vi "cliente_planta.vi"() -> ()   [LabVIEW 2023]
panel:
  in  "porta":dbl
  in  "agua cm3/s":dbl(slide) scale=0.0..500.0
  in  "barita g/s":dbl(slide) scale=0.0..1000.0
  out "DENSIDADE E SET POINT":cluster{dbl, "Setpoint":dbl}(graph)
  out "Numeric":dbl
  in  "ON/ OFF":bool
  out "DOSAGEM mA":string
  out "bytes escritos":i32
  out "corrente mA":string
  out "tipo de dosagem":string
  in  "Setpoint":dbl(slide) scale=0.8..1.4
  out "dado enviado para o servidor":string
  out "indicador de set point":string
  out "indicador de densidade":string
  in  "parametro a":dbl format="%#_13g"
  in  "parametro b":dbl format="%#_13g"
  in  "parametro c":dbl format="%#_13g"
  out "densidadeA":dbl
  out "SINAL DE CONTROLE AGUA":dbl(graph)
  out "Q1":dbl
  out "densidadeB":dbl
  out "SINAL DE CONTROLE BARITA":dbl(graph)
  in  "A":dbl=0.1 format="%#_13g"
  in  "B":dbl=0.2 format="%#_13g"
  in  "C":dbl format="%#_13g"
  out "W2":dbl
  # "MODELO/BARITA"
  # "MODELO/ÁGUA"
  # "SAÍDA DO CLIENTE/ENTRADA DO CONTROLADOR"
  # "SAÍDA DO SERVIDOR/AÇÃO DE CONTROLE"
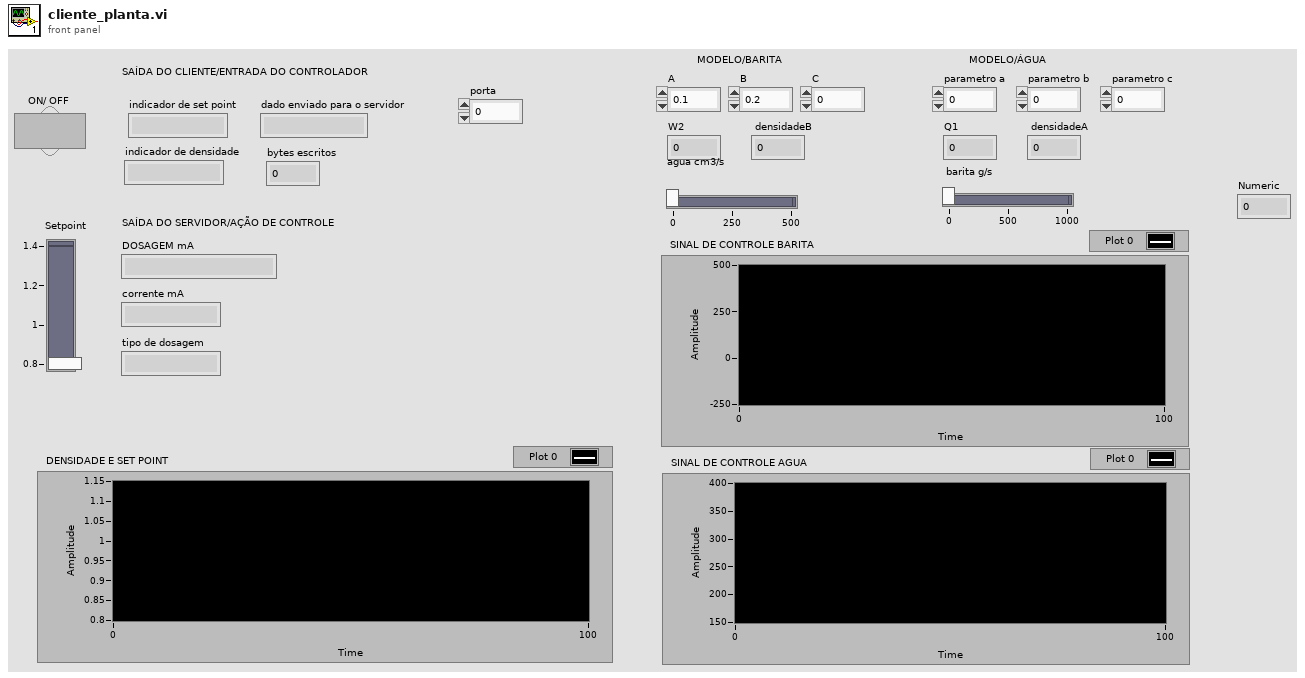
[diagram p1: front panel]
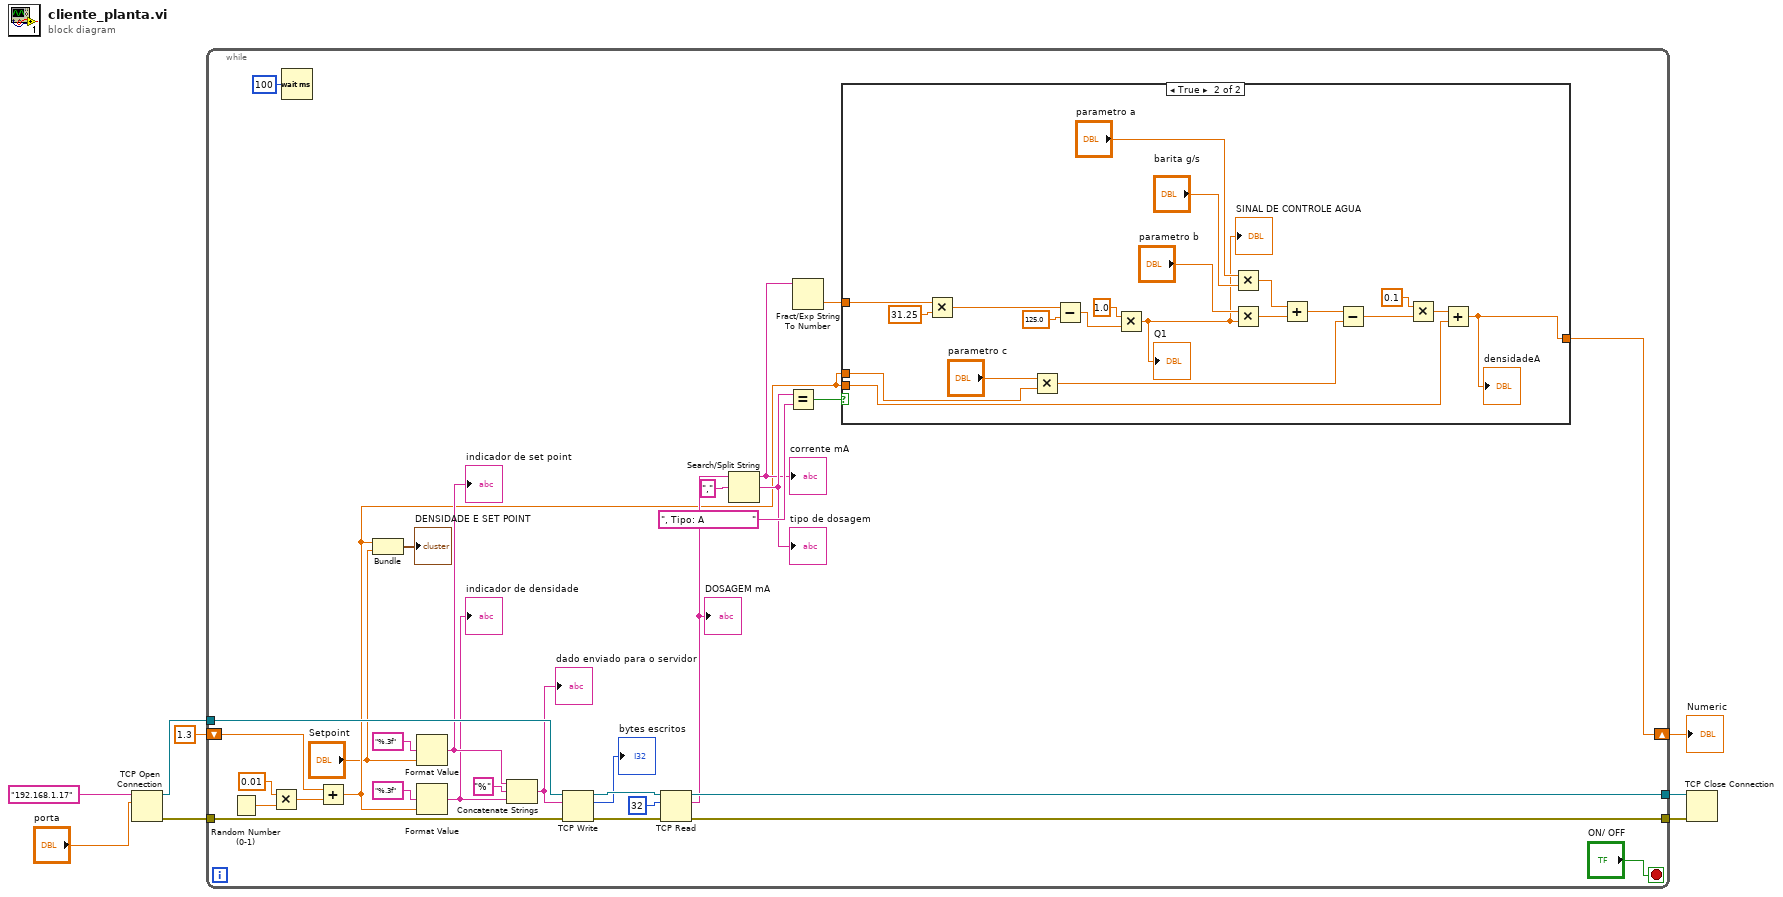
[diagram p0: block diagram]
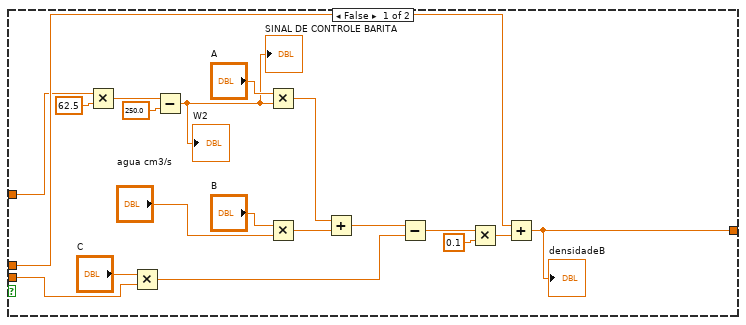
[diagram p2: hidden frame]
diagram:
  n1 = TCP Open Connection(address="192.168.1.17", remote port or service name="porta") -> (connection ID=w7:refnum<k5>, error out=w6:errorcluster)  [unwired: 3 in]
  n2 = while {
    tunnel: w7 -> [w37]
    tunnel: w6 -> [w36]
    tunnel: [w33] -> w5
    tunnel: [w32] -> w4
    shift-right: [w18] -> w2
    shift-left: 1.3 -> [w15]
    stop <- "ON/ OFF" stop-if-true
    n3 = Random Number (0-1)() -> (number: 0 to 1=w14:dbl)
    n4 = Multiply(x=0.01, y=w14) -> (x*y=w13:dbl)
    n5 = Wait (ms)(milliseconds to wait=100) -> ()  [unwired: 1 out]
    n6 = Add(x=w15, y=w13) -> (x+y=w11:dbl)
    n7 = Bundle(w11, "Setpoint"="Setpoint") -> (→"DENSIDADE E SET POINT":cluster{dbl, "Setpoint":dbl})  [unwired: 1 in]
    n8 = Format Value(format string="%.3f", value (0)="Setpoint") -> (output string=w22:string)  [unwired: 1 in]
    "indicador de set point" <- w22
    n9 = Format Value(format string="%.3f", value (0)=w11) -> (output string=w21:string)  [unwired: 1 in]
    "indicador de densidade" <- w21
    n10 = Concatenate Strings(w22, "%" ("string"), w21) -> (w25:string)
    "dado enviado para o servidor" <- w25
    n11 = TCP Write(connection ID=w37, data in=w25, error in (no error)=w36) -> (connection ID out=w35:refnum<k5>, bytes written=→"bytes escritos":i32, error out=w34:errorcluster)  [unwired: 1 in]
    n12 = TCP Read(connection ID=w35, bytes to read=32, error in (no error)=w34) -> (connection ID out=w32:refnum<k5>, data out=w29:string, error out=w33:errorcluster)  [unwired: 2 in]
    "DOSAGEM mA" <- w29
    n13 = Search/Split String(string=w29, search string/char (-)=",") -> (substring before match=w17:string, match + rest of string=w20:string)  [unwired: 1 in, 1 out]
    "corrente mA" <- w17
    "tipo de dosagem" <- w20
    n14 = Equal?(x=w20, y=", Tipo: A                ") -> (x = y?=w19:bool)
    n15 = Fract/Exp String To Number(string=w17) -> (number=w16:dbl)  [unwired: 3 in, 1 out]
    n16 = case shown="True" w19 {
      tunnel: [w52 w67] -> w18
      tunnel: w16 -> [w42 w66]
      tunnel: w11 -> [w49 w68]
      tunnel: w11 -> [w46 w74]
      frame False {
        n17 = Multiply(x=w42, y=62.5) -> (x*y=w44:dbl)
        n18 = Multiply(x="C", y=w49) -> (x*y=w48:dbl)
        n19 = Subtract(x=w44, y=250.0) -> (x-y=w41:dbl)
        "SINAL DE CONTROLE BARITA" <- w41
        "W2" <- w41
        n20 = Multiply(x="A", y=w41) -> (x*y=w54:dbl)
        n21 = Multiply(x="B", y="agua cm3/s") -> (x*y=w53:dbl)
        n22 = Add(x=w54, y=w53) -> (x+y=w51:dbl)
        n23 = Subtract(x=w51, y=w48) -> (x-y=w47:dbl)
        n24 = Multiply(x=w47, y=0.1) -> (x*y=w55:dbl)
        n25 = Add(x=w46, y=w55) -> (x+y=w52:dbl)
        "densidadeB" <- w52
      }
      frame True {
        n26 = Multiply(x=w66, y=31.25) -> (x*y=w64:dbl)
        n27 = Multiply(x="parametro c", y=w74) -> (x*y=w73:dbl)
        n28 = Subtract(x=w64, y=125.0) -> (x-y=w61:dbl)
        n29 = Multiply(x=1.0, y=w61) -> (x*y=w59:dbl)
        "SINAL DE CONTROLE AGUA" <- w59
        "Q1" <- w59
        n30 = Multiply(x="parametro a", y="barita g/s") -> (x*y=w77:dbl)
        n31 = Multiply(x="parametro b", y=w59) -> (x*y=w76:dbl)
        n32 = Add(x=w77, y=w76) -> (x+y=w72:dbl)
        n33 = Subtract(x=w72, y=w73) -> (x-y=w71:dbl)
        n34 = Multiply(x=0.1, y=w71) -> (x*y=w69:dbl)
        n35 = Add(x=w69, y=w68) -> (x+y=w67:dbl)
        "densidadeA" <- w67
      }
    }
  }
  "Numeric" <- w2
  n36 = TCP Close Connection(connection ID=w4, error in (no error)=w5) -> ()  [unwired: 1 in, 2 out]
